vi "Fault Handling.vi"(7 "Stop":refnum<user-event>, 8 "error in (no error)":errorcluster, 10 "FaultCode":i32, 11 "TestExec in":refnum<class "TestExec.lvclass">) -> (0 "error out":errorcluster, 3 "TestExec out":refnum<class "TestExec.lvclass">)   [LabVIEW 2021, in "TestExec.lvclass"]
uses:
  TestExec.lvclass
  TestExec.lvclass/TestExec.ctl
  <vilib>/addons/TestStand/_TSUtility.llb/TestStand - Set Property Value (Number).vi
  <vilib>/addons/TestStand/_TSUtility.llb/TestStand - Set Property Value (String).vi
  <vilib>/addons/TestStand/_TSUtility.llb/TestStand - Set Property Value (Boolean).vi
  OPC UA/OPC UA.lvclass
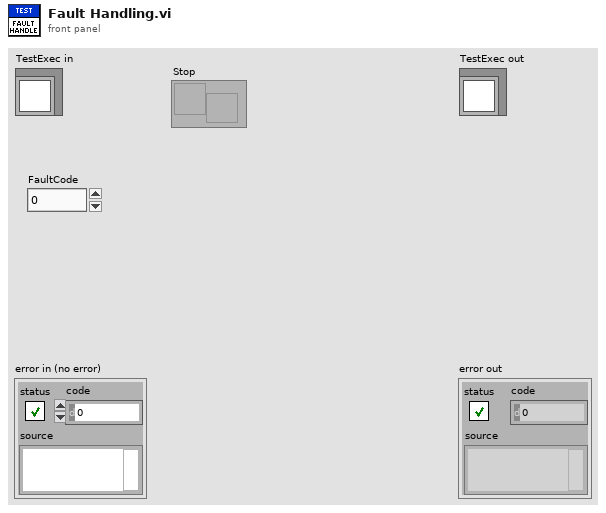
[diagram p1: front panel]
types:
  T1 = typedef "TestExec.lvclass/Rx TestExec.ctl" = cluster{"Cylinder_1":bool, "Cylinder_2":bool, "Cylinder_3":bool, "Cylinder_4":bool, "Cylinder_5":bool, "StepEcho":i32, "Reset":bool, "Stop":bool, "FaultCode":u32}
  T2 = typedef "TestExec.lvclass/Tx TestExec.ctl" = cluster{"HighVoltage":bool, "TestRunning":bool, "StepNo":i32, "Fault":bool}
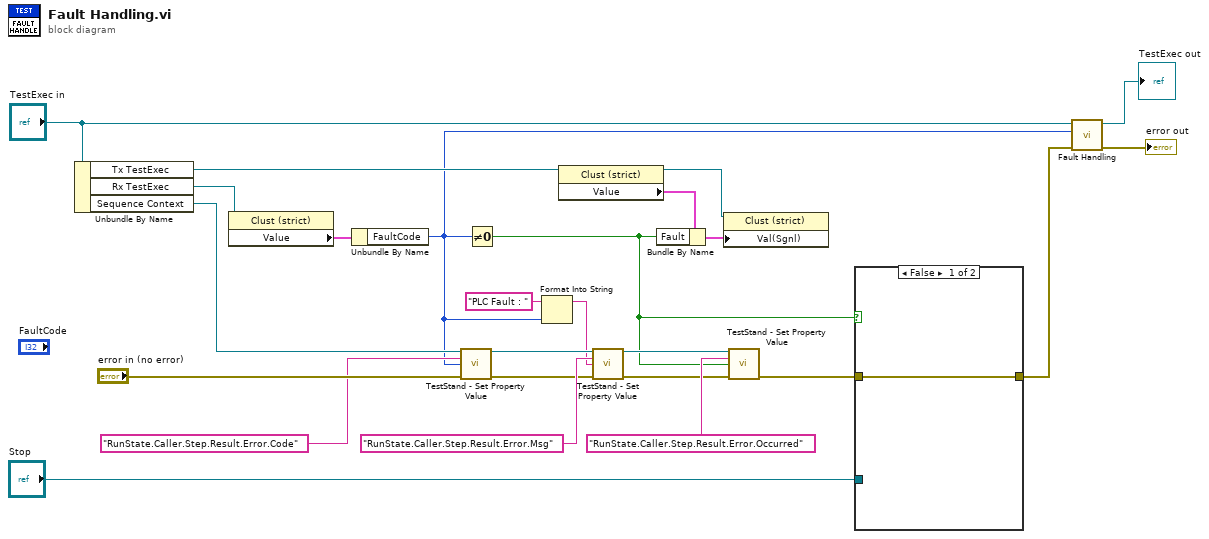
[diagram p0: block diagram]
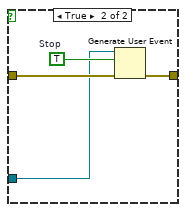
[diagram p2: hidden frame]
diagram:
  n1 = Unbundle By Name("TestExec in") -> ("Tx TestExec"=w22:refnum<vi>, "Rx TestExec"=w20:refnum<vi>, "Sequence Context"=w16:refnum<k7>)
  n2 = property class="Clust (strict)"(reference=w20) -> ("Value"=w21:T1)  [unwired: 1 in, 2 out]
  n3 = Unbundle By Name(w21) -> ("FaultCode"=w5:u32)
  n4 = call-poly <vilib>:"TestStand - Set Property Value.vi"("Sequence Context In"=w16, "Lookup String"="RunState.Caller.Step.Result.Error.Code", "New Value"=w5, "error in (no error)"="error in (no error)") -> ("Sequence Context Out"=w9:refnum<k7>, "error out"=w11:errorcluster)  [unwired: 10 in]
  n5 = Not Equal To 0?(x=w5) -> (x != 0?=w2:bool)
  n6 = Format Into String(initial string="PLC Fault : ", w5) -> (resulting string=w6:string)  [unwired: 2 in, 1 out]
  n7 = property class="Clust (strict)"(reference=w22) -> (reference out=w25:refnum<vi>, "Value"=w23:T2)  [unwired: 1 in, 1 out]
  n8 = call-poly <vilib>:"TestStand - Set Property Value.vi"("Sequence Context In"=w9, "Lookup String"="RunState.Caller.Step.Result.Error.Msg", "New Value"=w6, "error in (no error)"=w11) -> ("Sequence Context Out"=w8:refnum<k7>, "error out"=w10:errorcluster)  [unwired: 10 in]
  n9 = Bundle By Name(cluster=w23, "Fault"=w2) -> (w24:T2)
  n10 = property class="Clust (strict)"(reference=w25, "Val(Sgnl)"=w24) -> ()  [unwired: 1 in, 2 out]
  n11 = call-poly <vilib>:"TestStand - Set Property Value.vi"("Sequence Context In"=w8, "Lookup String"="RunState.Caller.Step.Result.Error.Occurred", "New Value"=w2, "error in (no error)"=w10) -> ("error out"=w4:errorcluster)  [unwired: 10 in, 1 out]
  n12 = case shown="False" w2 {
    tunnel: "Stop" -> [_ w27]
    tunnel: w4 -> [w26 w29]
    tunnel: [w26 w28] -> w3
    frame False {
    }
    frame True {
      w30 = TRUE  # Stop
      n13 = Generate User Event(user event=w27, event data cluster=w30, error in=w29) -> (error out=w28:errorcluster)  [unwired: 1 in, 1 out]
    }
  }
  n14 = call-parent "Fault Handling.vi"("error in (no error)"=w3, "FaultCode"=w5, "OPC UA in"="TestExec in") -> ("error out"=→"error out":errorcluster, "OPC UA out"=→"TestExec out":refnum<class "TestExec.lvclass">)  [unwired: 7 in]
